vi "LIA_FPGA.vi"() -> ()   [LabVIEW 2012]
uses:
  <vilib>/LabVIEW Targets/FPGA/cRIO/shared/nicrio_ModuleControls/nicrio_cRIO-9233_DataRatesRing.ctl
  <vilib>/rvi/DataTransferAndStorage/Container/Common/niFpgaContainerMetaDataKey.ctl
  <vilib>/rvi/DataTransferAndStorage/Container/Common/niFpgaContainerState.ctl
  <vilib>/rvi/DataTransferAndStorage/Container/Common/niFpgaDataTypeControl.ctl
  <vilib>/rvi/DataTransferAndStorage/Container/Common/niFpgaContainerImplementationControl.ctl
  <vilib>/rvi/DataTransferAndStorage/Container/Common/niFpgaContainerArbitrationOptionsControl.ctl
  <vilib>/rvi/DataTransferAndStorage/Container/Common/niFpgaTransferTypeControl.ctl
  <vilib>/rvi/DataTransferAndStorage/Container/Common/niFpgaContainerInitializationParameters.ctl
  <vilib>/rvi/Memory/Memory_Types/niFpgaMemoryInterfaceConfiguration.ctl
  <vilib>/rvi/FIFO/Fifo_Types/niFpgaFifoControlLogicControl.ctl
  <vilib>/Platform/TimedLoop/XDataNode/timing_clust.ctl
  <vilib>/Platform/TimedLoop/XDataNode/nitl_modes.ctl
  <vilib>/Platform/TimedLoop/XDataNode/wakeup.ctl
  <vilib>/rvi/FXPMathLib/FxpSinAndCos/subVIs/nifxpmath_SinAndCos_SimConfig.ctl
  <vilib>/rvi/DataTransferAndStorage/Container/Common/niFpgaContainerGetUniqueNameForEmu.vi
  <vilib>/rvi/DataTransferAndStorage/Container/Common/niFpgaContainerSetEmuInfo.vi
  <vilib>/rvi/eio/common/nirviEmuReportErrorAndStop.vi
  <vilib>/rvi/eio/common/nirviEmuTemplatePropertyGet_noerrors.vi
  <vilib>/rvi/eio/common/nirviEmuTemplatePropertySet_noerrors.vi
  <vilib>/rvi/eio/common/nirviEmuTemplateMethod_errors.vi
  <vilib>/rvi/FXPMathLib/FxpSinAndCos/simVIs/DllFxpSinAndCosTemp_sub.vi
  <vilib>/rvi/Emulation/niFpgaSctlEmulationGetInTimedLoop.vi
  <vilib>/rvi/FIFO/Fifo_Resource/nirvififoEmulationSetSize.vi
  <vilib>/rvi/errors/niFpgaSetErrorForExecOnDevCompSimple.vi
  <vilib>/rvi/Emulation/niFpgaSctlEmulationFifoFullMgr.vi
  <vilib>/rvi/Emulation/niFpgaSctlEmulationResourceMgr.vi
  <vilib>/rvi/interface/RandomDataEmulation/nirviRandomDataFPGAFIFO.vi
  <vilib>/rvi/interface/RandomDataEmulation/niFpgaRandomDataHandleErrors.vi
  <vilib>/rvi/Emulation/niFpgaSctlEmulationRegisterWithScheduler.vi
  <vilib>/rvi/Emulation/niFpgaSctlEmulationScheduler.vi
  <vilib>/rvi/LocalResourceManager/LocalResourceManager.xnode
  <vilib>/eio/EIOPropertyNode/EIOPropertyNode.xnode
  <vilib>/eio/EIONode/EIONode.xnode
  <vilib>/Platform/TimedLoop/XDataNode/XDataNode.xnode
  <vilib>/rvi/FXPMathLib/FxpSinAndCos/XNode/nifxpmath_SinAndCos.xnode
  <vilib>/rvi/DataTransferAndStorage/Container/XNode/niFpgaContainer.xnode
  <vilib>/rvi/FIFO/Fifo_Resource/nirvififoEmulationWrite.vi
  <vilib>/rvi/interface/RandomDataEmulation/nirviRandomDataFpgaReadWriteTemplate.vi
  <vilib>/rvi/FIFO/Fifo_Resource/nirvififoEmulationRead.vi
  <vilib>/Platform/TimedLoop/XDataNode/XDNodeRunTimeDep.lvlib
  <vilib>/rvi/eio/common/nirviEmuTemplatePropertyGet_errors.vi
  <vilib>/rvi/eio/common/nirviEmuTemplatePropertySet_errors.vi
panel:
  in  "dec":i32
  out "channelQ":i64
  out "channelI":i64
  in  "reset":bool
  in  "Data Rate":T1=2 items=["50.000 kS/s (NI 9233)"=2, "33.333 kS/s (NI 9233)"=3, "25.000 kS/s (NI 9233)"=34, "16.667 kS/s (NI 9233)"=35, "12.500 kS/s (NI 9233)"=36, "10.000 kS/s (NI 9233)"=37, "  8.333 kS/s (NI 9233)"=38, "  7.143 kS/s (NI 9233)"=39, "  6.250 kS/s (NI 9233)"=40, "  5.556 kS/s (NI 9233)"=41, "  5.000 kS/s (NI 9233)"=42, "  4.545 kS/s (NI 9233)"=43, "  4.167 kS/s (NI 9233)"=44, "  3.846 kS/s (NI 9233)"=45, "  3.571 kS/s (NI 9233)"=46, "  3.333 kS/s (NI 9233)"=47, "  3.125 kS/s (NI 9233)"=48, "  2.941 kS/s (NI 9233)"=49, "  2.778 kS/s (NI 9233)"=50, "  2.632 kS/s (NI 9233)"=51, "  2.500 kS/s (NI 9233)"=52, "  2.381 kS/s (NI 9233)"=53, "  2.273 kS/s (NI 9233)"=54, "  2.174 kS/s (NI 9233)"=55, "  2.083 kS/s (NI 9233)"=56, "  2.000 kS/s (NI 9233)"=57]
  out "f_2":fxp<+/-,32,0> format="%.32g"
  out "f":fxp<+/-,32,0> format="%.32g"
  out "Offset":i32
  out "LSB Weight":u32
  in  "channel":i16
  in  "test":bool
  out "error":bool
  in  "dec2":i16
  in  "K":fxp<+/-,16,1>
  in  "nominal freq":fxp<+/-,16,1>
  in  "dec1":i16
  in  "stages":i8=1
  in  "stop":bool
  in  "decimation":i16=1024
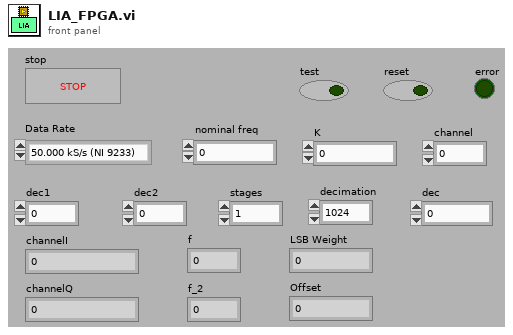
[diagram p1: front panel]
types:
  T1 = typedef "nicrio_cRIO-9233_DataRatesRing.ctl" = u8
  T2 = typedef "XDNodeRunTimeDep.lvlib/timing_clust.ctl" = cluster{"Expected End [f-1]":u64, "Actual End [f-1]":u64, "Finished Late? [f-1]":bool, "Expected End [i-1]":u64, "Actual End [i-1]":u64, "Finished Late? [i-1]":bool, "Expected Start [i]":u64, "Actual Start [i]":u64, "Expected Start [f]":u64, "Actual Start [f]":u64, "Source Name":string, "Structure Name":string, "Period":i64, "Deadline":i64, "Offset":i64, "Start":i64, "Priority":i32, "Timeout":i32, "Mode":T3, "Wakeup Reason":T4, "Error":errorcluster, "Source Type":string, "Secondary Source Type":string, "Global End Time":u64, "Global Start Time":u64, "Frame Duration":u64, "Iteration Duration":u64, "Assigned CPU":i32, "I/O Scan Engine Mode":u32}
  T3 = typedef "XDNodeRunTimeDep.lvlib/nitl_modes.ctl" = enum32{"No Change", "Process missed periods, maintain original phase", "Discard missed periods, maintain original phase", "Process missed periods, ignore original phase", "Discard missed periods, ignore original phase"}
  T4 = typedef "XDNodeRunTimeDep.lvlib/wakeup.ctl" = enum32{"Normal", "Aborted", "Asynchronous wakeup", "Timing source error", "Timed loop error", "Timeout"}
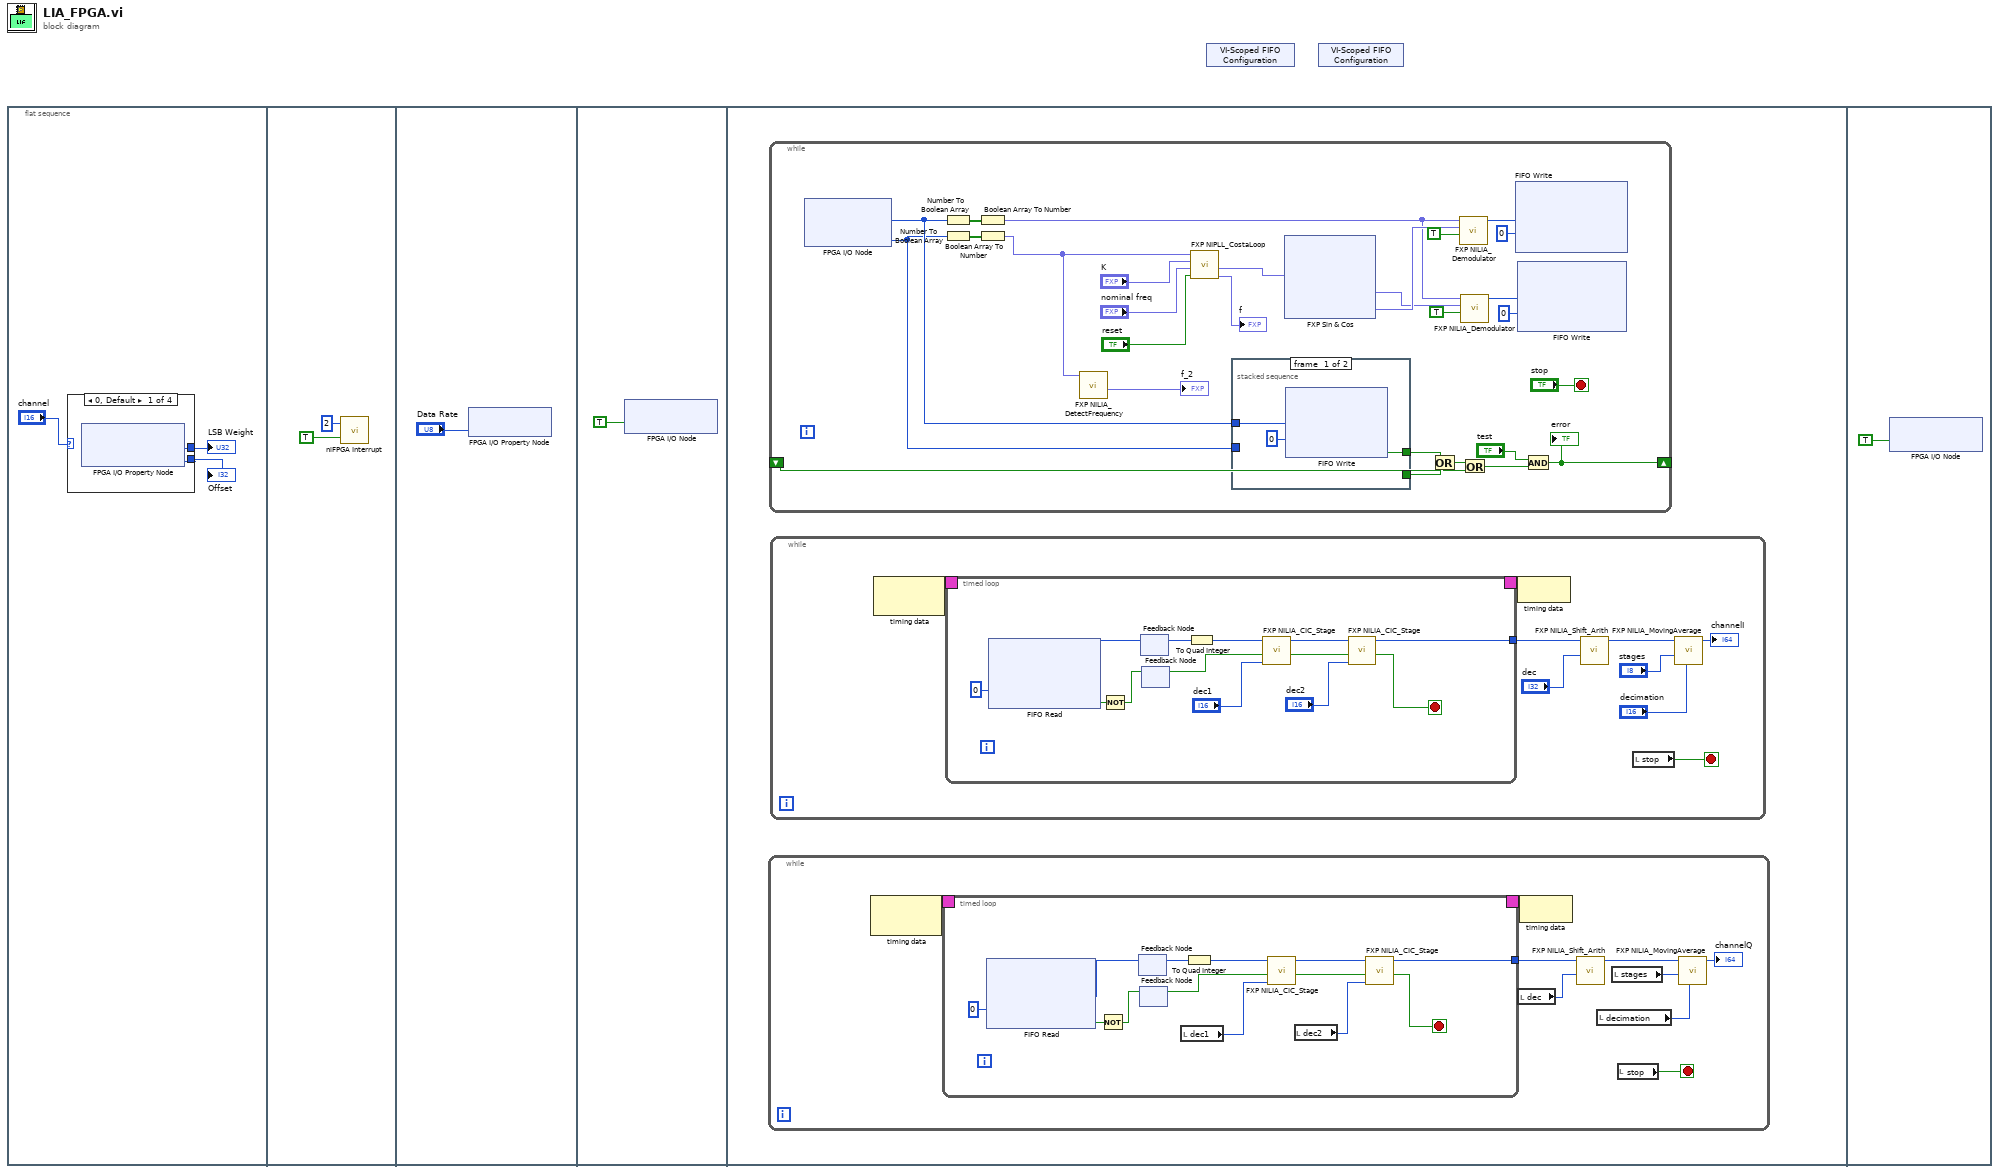
[diagram p0: block diagram]
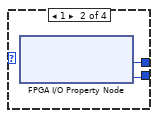
[diagram p2: hidden frame]
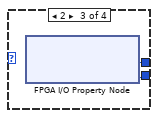
[diagram p3: hidden frame]
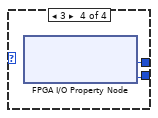
[diagram p4: hidden frame]
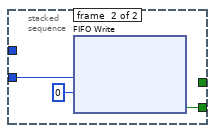
[diagram p5: hidden frame]
diagram:
  n1 = flat-sequence {
    frame #0 {
      n2 = case shown="0, Default" "channel" {
        tunnel: [w5 w7 w9 w11] -> w2
        tunnel: [w4 w6 w8 w10] -> w1
        frame 0, Default {
          n3 = xnode "FPGA I/O Property Node"() -> ("LSB Weight"=w5:u32, "Offset"=w4:i32)  [unwired: 1 in, 1 out]
        }
        frame 1 {
          n4 = xnode "FPGA I/O Property Node"() -> ("LSB Weight"=w7:u32, "Offset"=w6:i32)  [unwired: 1 in, 1 out]
        }
        frame 2 {
          n5 = xnode "FPGA I/O Property Node"() -> ("LSB Weight"=w9:u32, "Offset"=w8:i32)  [unwired: 1 in, 1 out]
        }
        frame 3 {
          n6 = xnode "FPGA I/O Property Node"() -> ("LSB Weight"=w11:u32, "Offset"=w10:i32)  [unwired: 1 in, 1 out]
        }
      }
      "LSB Weight" <- w2
      "Offset" <- w1
    }
    frame #1 {
      n7 = call <vilib>:"niFPGA Interrupt.vi"("Wait Until Cleared (F)"=TRUE ("Wait Until Cleared"), "IRQ Number (0)"=u8 2 ("IRQ Number")) -> ()  [unwired: 1 in]
    }
    frame #2 {
      n8 = xnode "FPGA I/O Property Node"("Data Rate"="Data Rate") -> ()  [unwired: 1 in, 1 out]
    }
    frame #3 {
      n9 = xnode "FPGA I/O Node"("Mod1/Start"=TRUE) -> ()  [unwired: 1 in, 1 out]
    }
    frame #4 {
      n10 = while {
        stop <- w22 stop-if-true
        n11 = node-c288() -> (w24:T2)  [unwired: 1 in]
        n12 = timed-loop {
          timing: w24 -> [_]
          timing-out: [_] -> w23
          tunnel: [w26] -> w21
          stop <- w25 stop-if-true
          n13 = xnode ("FIFO Read")("Timeout"=0) -> ("Element"=w35:i32, "Timed Out?"=w34:bool)  [unwired: 1 in, 1 out]
          n14 = Not(x=w34) -> (.not. x?=w33:bool)
          n15 = feedback-in #1(w35) -> ()
          n16 = feedback #1() -> (w37:i32)  [unwired: 1 in]
          n17 = feedback-in #2(w33) -> ()
          n18 = feedback #2() -> (w31:bool)  [unwired: 1 in]
          n19 = local read "dec1"() -> (w30:i16)
          n20 = To Quad Integer(1:w37) -> (0:w32:i64)
          n21 = call "FXP NILIA_CIC_Stage.vi"("decimate factor"=w30, "New Data"=w31, "input"=w32) -> ("Data Ready"=w28:bool, "output"=w29:i64)  [unwired: 7 in]
          n22 = local read "dec2"() -> (w27:i16)
          n23 = call "FXP NILIA_CIC_Stage.vi"("decimate factor"=w27, "New Data"=w28, "input"=w29) -> ("Data Ready"=w25:bool, "output"=w26:i64)  [unwired: 7 in]
        }
        n24 = local read "dec"() -> (w20:i32)
        n25 = node-c288(w23) -> ()
        n26 = call "FXP NILIA_Shift_Arith.vi"("dec"=w20, "x"=w21) -> ("y"=w19:i64)  [unwired: 9 in]
        n27 = local read "decimation"() -> (w17:i16)
        n28 = local read "stages"() -> (w18:i8)
        n29 = local read "stop"() -> (w22:bool)
        n30 = call "FXP NILIA_MovingAverage.vi"("decimate"=w17, "stages"=w18, "input"=w19) -> ("output"=→"channelQ":i64)  [unwired: 8 in]
      }
      n31 = while {
        shift-right: [w61] -> _
        shift-left: _ -> [w63]
        stop <- "stop" stop-if-true
        n32 = xnode "FPGA I/O Node"() -> ("Mod1/AI0"=w52:i32, "Mod1/AI1"=w51:i32)  [unwired: 2 in, 2 out]
        n33 = Number To Boolean Array(number=w52) -> (Boolean array=w54:bool[])
        n34 = Number To Boolean Array(number=w51) -> (Boolean array=w53:bool[])
        n35 = Boolean Array To Number(Boolean array=w54) -> (number=w45:fxp<+/-,24,1>)
        n36 = Boolean Array To Number(Boolean array=w53) -> (number=w50:fxp<+/-,24,1>)
        n37 = call "FXP NILIA_DetectFrequency.vi"("x"=w50) -> ("f_2"=→"f_2":fxp<+/-,32,0>)  [unwired: 9 in, 1 out]
        n38 = call "FXP NIPLL_CostaLoop.vi"("reset?"="reset", "norminal freq [U16.0]"="nominal freq", "alpha [U16.0]"="K", "x[I24.1]"=w50) -> ("f"=→"f":fxp<+/-,32,0>, "z [I32.1]"=w58:fxp<+/-,32,1>)  [unwired: 4 in, 2 out]
        n39 = stacked-sequence {
          tunnel: w52 -> [w101 _]
          tunnel: w51 -> [_ w104]
          tunnel: [w100 _] -> w67
          tunnel: [_ w103] -> w66
          frame #0 {
            n40 = xnode ("FIFO Write")("Element"=w101, "Timeout"=0) -> ("Timed Out?"=w100:bool)  [unwired: 1 in, 1 out]
          }
          frame #1 {
            n41 = xnode ("FIFO Write")("Element"=w104, "Timeout"=0) -> ("Timed Out?"=w103:bool)  [unwired: 1 in, 1 out]
          }
        }
        n42 = xnode "FXP Sin & Cos"("x (pi)"=w58) -> ("sin(x)"=w44:fxp<+/-,24,2>, "cos(x)"=w48:fxp<+/-,24,2>)
        n43 = Or(x=w67, y=w66) -> (x .or. y?=w65:bool)
        n44 = call "FXP NILIA_Demodulator.vi"("New Data"=TRUE, "ref"=w48, "signal"=w45) -> ("x*y"=w46:i32)  [unwired: 7 in, 1 out]
        n45 = call "FXP NILIA_Demodulator.vi"("New Data"=TRUE, "ref"=w44, "signal"=w45) -> ("x*y"=w42:i32)  [unwired: 7 in, 1 out]
        n46 = Or(x=w65, y=w63) -> (x .or. y?=w64:bool)
        n47 = xnode ("FIFO Write")("Element"=w46, "Timeout"=0) -> ()  [unwired: 1 in, 2 out]
        n48 = xnode ("FIFO Write")("Element"=w42, "Timeout"=0) -> ()  [unwired: 1 in, 2 out]
        n49 = And(x="test", y=w64) -> (x .and. y?=w61:bool)
        "error" <- w61
      }
      n50 = while {
        stop <- w112 stop-if-true
        n51 = node-c288() -> (w114:T2)  [unwired: 1 in]
        n52 = timed-loop {
          timing: w114 -> [_]
          timing-out: [_] -> w113
          tunnel: [w116] -> w111
          stop <- w115 stop-if-true
          n53 = xnode ("FIFO Read")("Timeout"=0) -> ("Element"=w125:i32, "Timed Out?"=w124:bool)  [unwired: 1 in, 1 out]
          n54 = Not(x=w124) -> (.not. x?=w123:bool)
          n55 = feedback-in #3(w125) -> ()
          n56 = feedback #3() -> (w127:i32)  [unwired: 1 in]
          n57 = feedback-in #4(w123) -> ()
          n58 = feedback #4() -> (w121:bool)  [unwired: 1 in]
          n59 = To Quad Integer(1:w127) -> (0:w122:i64)
          n60 = call "FXP NILIA_CIC_Stage.vi"("decimate factor"="dec1", "New Data"=w121, "input"=w122) -> ("Data Ready"=w118:bool, "output"=w119:i64)  [unwired: 7 in]
          n61 = call "FXP NILIA_CIC_Stage.vi"("decimate factor"="dec2", "New Data"=w118, "input"=w119) -> ("Data Ready"=w115:bool, "output"=w116:i64)  [unwired: 7 in]
        }
        n62 = node-c288(w113) -> ()
        n63 = call "FXP NILIA_Shift_Arith.vi"("dec"="dec", "x"=w111) -> ("y"=w109:i64)  [unwired: 9 in]
        n64 = local read "stop"() -> (w112:bool)
        n65 = call "FXP NILIA_MovingAverage.vi"("decimate"="decimation", "stages"="stages", "input"=w109) -> ("output"=→"channelI":i64)  [unwired: 8 in]
      }
    }
    frame #5 {
      n66 = xnode "FPGA I/O Node"("Mod1/Stop"=TRUE) -> ()  [unwired: 1 in, 1 out]
    }
  }
  n67 = xnode "VI-Scoped FIFO Configuration"() -> ()  [unwired: 1 out]
  n68 = xnode "VI-Scoped FIFO Configuration"() -> ()  [unwired: 1 out]
